vi "fleep fplap.vi"(1 "False":bool, 2 "True":bool) -> (0 "State":bool)   [LabVIEW 2014]
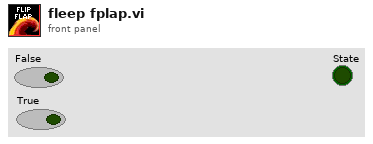
[diagram p1: front panel]
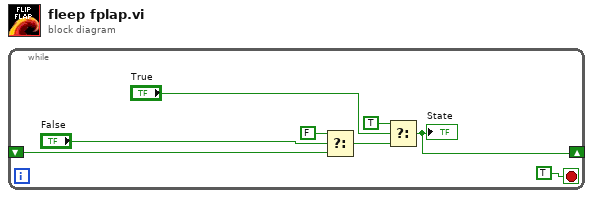
[diagram p0: block diagram]
diagram:
  n1 = while {
    shift-right: [w5] -> _
    shift-left: _ -> [w4]
    stop <- TRUE stop-if-true
    n2 = Select(t=FALSE, s="False", f=w4) -> (s? t:f=w1:bool)
    n3 = Select(t=TRUE, s="True", f=w1) -> (s? t:f=w5:bool)
    "State" <- w5
  }
